vi "_Validate Active Channels.vi"(4 "Negative (F)":bool, 5 "Resolution Type":T1 items=["High/High", "Medium/Medium", "Low/Low", "High/Medium", "High/Low", "Medium/High", "Medium/Low", "Low/High", "Low/Medium"], 6 "error in":errorcluster, 7 "Expt#":i32, 8 "User Res Table (T)":bool=TRUE, 9 "Active Ch":T2[](array[typedef])) -> (0 "error out":errorcluster, 2 "DAC Values":i32[](array[numeric]), 3 "Ch ID":i32[](array[numeric]))   [LabVIEW 2012]
uses:
  Type/_RT Active Ch.ctl
  Type/_RT Res Type.ctl
  _RT Global.vi
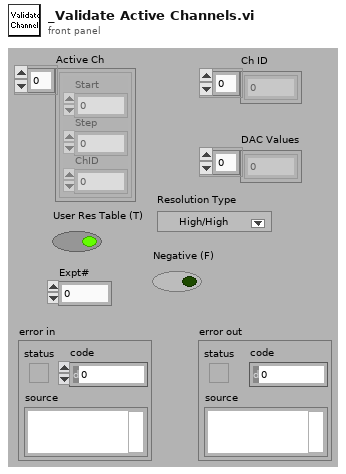
[diagram p1: front panel]
types:
  T1 = typedef "_RT Res Type.ctl" = u16
  T2 = typedef "_RT Active Ch.ctl" = cluster{"Start":i32, "Step":i32, "ChID":i32}
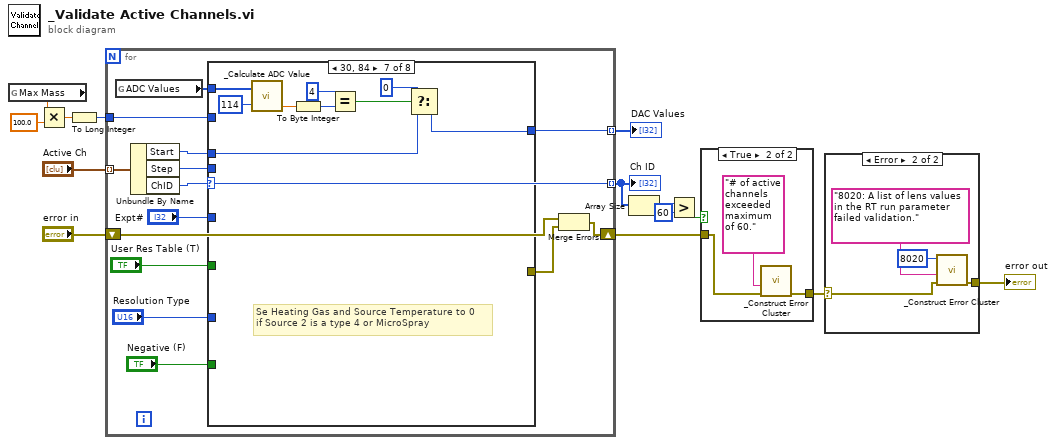
[diagram p0: block diagram]
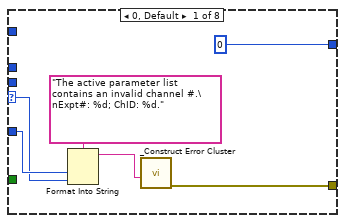
[diagram p4: hidden frame]
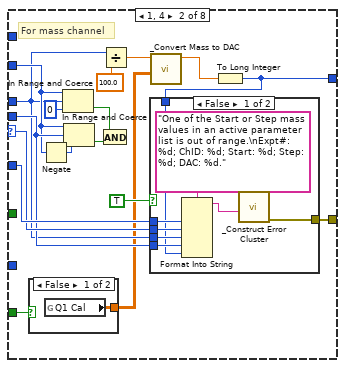
[diagram p5: hidden frame]
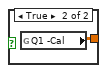
[diagram p6: hidden frame]
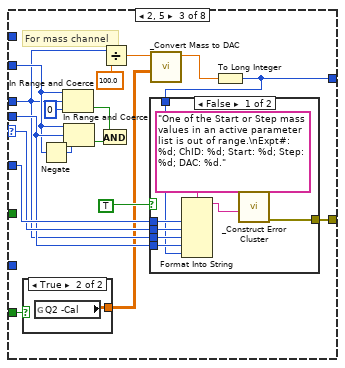
[diagram p8: hidden frame]
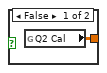
[diagram p9: hidden frame]
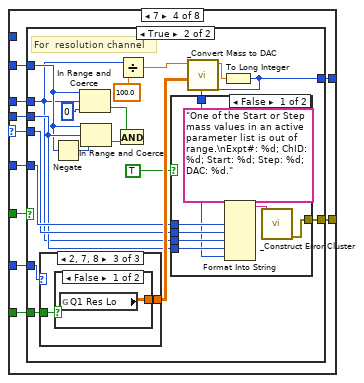
[diagram p11: hidden frame]
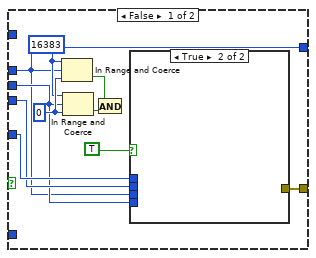
[diagram p12: hidden frame]
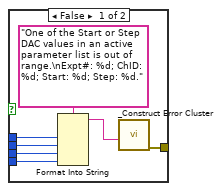
[diagram p13: hidden frame]
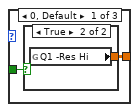
[diagram p14: hidden frame]
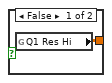
[diagram p15: hidden frame]
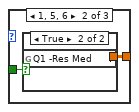
[diagram p16: hidden frame]
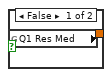
[diagram p17: hidden frame]
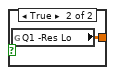
[diagram p18: hidden frame]
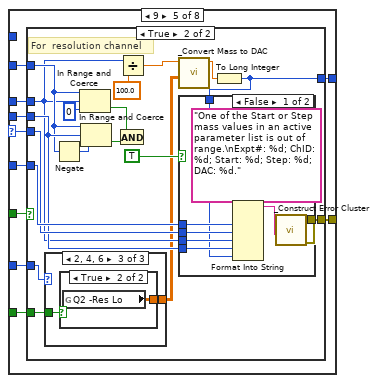
[diagram p20: hidden frame]
diagram:
  n1 = global read "_RT Global.vi" "Max Mass"() -> (w12:dbl)
  n2 = Multiply(x=w12, y=100.0) -> (x*y=w10:dbl)
  n3 = To Long Integer(number=w10) -> (32bit integer=w9:i32)
  n4 = for {
    tunnel: "Active Ch" -> [w28] mode=indexing
    shift-right: [w24] -> w3
    shift-left: "error in" -> [w23]
    tunnel: w9 -> [w25]
    tunnel: [w21] -> w7 mode=indexing
    tunnel: [w20] -> w8 mode=indexing
    n5 = global read "_RT Global.vi" "ADC Values"() -> (w15:i32[])
    n6 = Unbundle By Name(w28) -> ("Start"=w27:i32, "Step"=w26:i32, "ChID"=w21:i32)
    n7 = case shown="30, 84" w21 {
      selector: w21 -> [w31 w43 w70 w91 w156 _ _ w242]
      tunnel: [w34 w48 w75 w93 w158 _ _ w245] -> w22
      tunnel: w27 -> [_ w37 w65 w98 w163 w220 w229 w237]
      tunnel: w26 -> [_ w42 w69 w96 w161 _ _ w241]
      tunnel: w25 -> [_ w38 w67 w97 w162 _ _ _]
      tunnel: [0 ("lower limit") w41 w68 w95 w160 w219 w228 w237] -> w20
      tunnel: "User Res Table (T)" -> [_ _ _ w94 w159 _ _ _]
      tunnel: "Expt#" -> [w32 w44 w71 w92 w157 _ _ w243]
      tunnel: "Resolution Type" -> [_ _ _ w90 w155 _ _ _]
      tunnel: "Negative (F)" -> [_ w36 w63 w89 w154 _ _ _]
      tunnel: w15 -> [_ _ _ _ _ w227 w236 _]
      frame 0, Default {
        n8 = Format Into String(format string="The active parameter list contains an invalid channel #.\nExpt#: %d; ChID: %d.", w32, w31) -> (resulting string=w29:string)  [unwired: 2 in, 1 out]
        n9 = call "_Construct Error Cluster.vi"("reason"=w29) -> ("error out"=w34:errorcluster)  [unwired: 3 in, 3 out]
      }
      frame 1, 4 {
        # "For mass channel"
        n10 = case shown="False" w36 {
          tunnel: [w52 w53] -> w35
          frame False {
            n11 = global read "_RT Global.vi" "Q1 Cal"() -> (w52:dbl[][])
          }
          frame True {
            n12 = global read "_RT Global.vi" "Q1 -Cal"() -> (w53:dbl[][])
          }
        }
        n13 = Negate(x=w38) -> (-x=w40:i32)
        n14 = In Range and Coerce(upper limit=w38, x=w37, lower limit=0) -> (In Range?=w50:bool)  [unwired: 1 out]
        n15 = In Range and Coerce(upper limit=w38, x=w42, lower limit=w40) -> (In Range?=w49:bool)  [unwired: 1 out]
        n16 = And(x=w50, y=w49) -> ()  [unwired: 1 out]
        n17 = Divide(x=w37, y=100.0) -> (x/y=w46:dbl)
        n18 = call "_Convert Mass to DAC.vi"("Calibration Table"=w35, "Mass"=w46) -> ("DAC Value"=w45:dbl)  [unwired: 2 in, 3 out]
        n19 = To Long Integer(number=w45) -> (32bit integer=w41:i32)
        n20 = case shown="False" TRUE {
          tunnel: [w61 _] -> w48
          tunnel: w44 -> [w59 _]
          tunnel: w43 -> [w58 _]
          tunnel: w37 -> [w57 _]
          tunnel: w42 -> [w56 _]
          tunnel: w41 -> [w54 _]
          frame False {
            n21 = Format Into String(format string="One of the Start or Step mass values in an active parameter list is out of range.\nExpt#: %d; ChID: %d; Start: %d; Step: %d; DAC: %d.", w59, w58, w57, w56, w54) -> (resulting string=w55:string)  [unwired: 2 in, 1 out]
            n22 = call "_Construct Error Cluster.vi"("reason"=w55) -> ("error out"=w61:errorcluster)  [unwired: 3 in, 3 out]
          }
          frame True {
          }
        }
      }
      frame 2, 5 {
        # "For mass channel"
        n23 = case shown="True" w63 {
          tunnel: [w79 w80] -> w62
          frame False {
            n24 = global read "_RT Global.vi" "Q2 Cal"() -> (w79:dbl[][])
          }
          frame True {
            n25 = global read "_RT Global.vi" "Q2 -Cal"() -> (w80:dbl[][])
          }
        }
        n26 = Negate(x=w67) -> (-x=w66:i32)
        n27 = In Range and Coerce(upper limit=w67, x=w65, lower limit=0) -> (In Range?=w77:bool)  [unwired: 1 out]
        n28 = In Range and Coerce(upper limit=w67, x=w69, lower limit=w66) -> (In Range?=w76:bool)  [unwired: 1 out]
        n29 = And(x=w77, y=w76) -> ()  [unwired: 1 out]
        n30 = Divide(x=w65, y=100.0) -> (x/y=w73:dbl)
        n31 = call "_Convert Mass to DAC.vi"("Calibration Table"=w62, "Mass"=w73) -> ("DAC Value"=w72:dbl)  [unwired: 2 in, 3 out]
        n32 = To Long Integer(number=w72) -> (32bit integer=w68:i32)
        n33 = case shown="False" TRUE {
          tunnel: [w88 _] -> w75
          tunnel: w71 -> [w86 _]
          tunnel: w70 -> [w85 _]
          tunnel: w65 -> [w84 _]
          tunnel: w69 -> [w83 _]
          tunnel: w68 -> [w81 _]
          frame False {
            n34 = Format Into String(format string="One of the Start or Step mass values in an active parameter list is out of range.\nExpt#: %d; ChID: %d; Start: %d; Step: %d; DAC: %d.", w86, w85, w84, w83, w81) -> (resulting string=w82:string)  [unwired: 2 in, 1 out]
            n35 = call "_Construct Error Cluster.vi"("reason"=w82) -> ("error out"=w88:errorcluster)  [unwired: 3 in, 3 out]
          }
          frame True {
          }
        }
      }
      frame 7 {
        n36 = case shown="True" w94 {
          tunnel: w98 -> [w99 w119]
          tunnel: w97 -> [_ w120]
          tunnel: w96 -> [w101 w123]
          tunnel: [w99 w122] -> w95
          tunnel: [w104 w126] -> w93
          tunnel: w92 -> [w103 w125]
          tunnel: w91 -> [w102 w124]
          tunnel: w90 -> [_ w117]
          tunnel: w89 -> [_ w116]
          frame False {
            w105 = 16383 ("lower limit")
            w108 = 0 ("lower limit")
            n37 = In Range and Coerce(upper limit=w105, x=w99, lower limit=w108) -> (In Range?=w107:bool)  [unwired: 1 out]
            n38 = In Range and Coerce(upper limit=w105, x=w101, lower limit=w108) -> (In Range?=w106:bool)  [unwired: 1 out]
            n39 = And(x=w107, y=w106) -> ()  [unwired: 1 out]
            n40 = case shown="True" TRUE {
              tunnel: [w115 _] -> w104
              tunnel: w103 -> [w114 _]
              tunnel: w102 -> [w113 _]
              tunnel: w99 -> [w112 _]
              tunnel: w101 -> [w111 _]
              frame False {
                n41 = Format Into String(format string="One of the Start or Step  DAC values in an active parameter list is out of range.\nExpt#: %d; ChID: %d; Start: %d; Step: %d.", w114, w113, w112, w111) -> (resulting string=w109:string)  [unwired: 2 in, 1 out]
                n42 = call "_Construct Error Cluster.vi"("reason"=w109) -> ("error out"=w115:errorcluster)  [unwired: 3 in, 3 out]
              }
              frame True {
              }
            }
          }
          frame True {
            # "For  resolution channel"
            n43 = case shown="2, 7, 8" w117 {
              tunnel: [w135 w139 w143] -> w130
              tunnel: w116 -> [w134 w138 w142]
              frame 0, Default {
                n44 = case shown="True" w134 {
                  tunnel: [w136 w137] -> w135
                  frame False {
                    n45 = global read "_RT Global.vi" "Q1 Res Hi"() -> (w136:dbl[][])
                  }
                  frame True {
                    n46 = global read "_RT Global.vi" "Q1 -Res Hi"() -> (w137:dbl[][])
                  }
                }
              }
              frame 1, 5, 6 {
                n47 = case shown="True" w138 {
                  tunnel: [w140 w141] -> w139
                  frame False {
                    n48 = global read "_RT Global.vi" "Q1 Res Med"() -> (w140:dbl[][])
                  }
                  frame True {
                    n49 = global read "_RT Global.vi" "Q1 -Res Med"() -> (w141:dbl[][])
                  }
                }
              }
              frame 2, 7, 8 {
                n50 = case shown="False" w142 {
                  tunnel: [w144 w145] -> w143
                  frame False {
                    n51 = global read "_RT Global.vi" "Q1 Res Lo"() -> (w144:dbl[][])
                  }
                  frame True {
                    n52 = global read "_RT Global.vi" "Q1 -Res Lo"() -> (w145:dbl[][])
                  }
                }
              }
            }
            n53 = Negate(x=w120) -> (-x=w121:i32)
            n54 = In Range and Coerce(upper limit=w120, x=w119, lower limit=0) -> (In Range?=w132:bool)  [unwired: 1 out]
            n55 = In Range and Coerce(upper limit=w120, x=w123, lower limit=w121) -> (In Range?=w131:bool)  [unwired: 1 out]
            n56 = And(x=w132, y=w131) -> ()  [unwired: 1 out]
            n57 = Divide(x=w119, y=100.0) -> (x/y=w128:dbl)
            n58 = call "_Convert Mass to DAC.vi"("Calibration Table"=w130, "Mass"=w128) -> ("DAC Value"=w127:dbl)  [unwired: 2 in, 3 out]
            n59 = To Long Integer(number=w127) -> (32bit integer=w122:i32)
            n60 = case shown="False" TRUE {
              tunnel: [w153 _] -> w126
              tunnel: w125 -> [w151 _]
              tunnel: w124 -> [w150 _]
              tunnel: w119 -> [w149 _]
              tunnel: w123 -> [w148 _]
              tunnel: w122 -> [w146 _]
              frame False {
                n61 = Format Into String(format string="One of the Start or Step mass values in an active parameter list is out of range.\nExpt#: %d; ChID: %d; Start: %d; Step: %d; DAC: %d.", w151, w150, w149, w148, w146) -> (resulting string=w147:string)  [unwired: 2 in, 1 out]
                n62 = call "_Construct Error Cluster.vi"("reason"=w147) -> ("error out"=w153:errorcluster)  [unwired: 3 in, 3 out]
              }
              frame True {
              }
            }
          }
        }
      }
      frame 9 {
        n63 = case shown="True" w159 {
          tunnel: w163 -> [w164 w185]
          tunnel: w162 -> [_ w186]
          tunnel: w161 -> [w166 w189]
          tunnel: [w164 w188] -> w160
          tunnel: [w169 w192] -> w158
          tunnel: w157 -> [w168 w191]
          tunnel: w156 -> [w167 w190]
          tunnel: w155 -> [_ w183]
          tunnel: w154 -> [_ w182]
          frame False {
            w170 = 16383 ("lower limit")
            w173 = 0 ("lower limit")
            n64 = In Range and Coerce(upper limit=w170, x=w164, lower limit=w173) -> (In Range?=w172:bool)  [unwired: 1 out]
            n65 = In Range and Coerce(upper limit=w170, x=w166, lower limit=w173) -> (In Range?=w171:bool)  [unwired: 1 out]
            n66 = And(x=w172, y=w171) -> ()  [unwired: 1 out]
            n67 = case shown="True" TRUE {
              tunnel: [w180 _] -> w169
              tunnel: w168 -> [w179 _]
              tunnel: w167 -> [w178 _]
              tunnel: w164 -> [w177 _]
              tunnel: w166 -> [w176 _]
              frame False {
                n68 = Format Into String(format string="One of the Start or Step  DAC values in an active parameter list is out of range.\nExpt#: %d; ChID: %d; Start: %d; Step: %d.", w179, w178, w177, w176) -> (resulting string=w174:string)  [unwired: 2 in, 1 out]
                n69 = call "_Construct Error Cluster.vi"("reason"=w174) -> ("error out"=w180:errorcluster)  [unwired: 3 in, 3 out]
              }
              frame True {
              }
            }
          }
          frame True {
            # "For  resolution channel"
            n70 = case shown="2, 4, 6" w183 {
              tunnel: [w200 w204 w208] -> w181
              tunnel: w182 -> [w199 w203 w207]
              frame 0, Default {
                n71 = case shown="False" w199 {
                  tunnel: [w201 w202] -> w200
                  frame False {
                    n72 = global read "_RT Global.vi" "Q2 Res Hi"() -> (w201:dbl[][])
                  }
                  frame True {
                    n73 = global read "_RT Global.vi" "Q2 -Res Hi"() -> (w202:dbl[][])
                  }
                }
              }
              frame 1, 3, 8 {
                n74 = case shown="False" w203 {
                  tunnel: [w205 w206] -> w204
                  frame False {
                    n75 = global read "_RT Global.vi" "Q2 Res Med"() -> (w205:dbl[][])
                  }
                  frame True {
                    n76 = global read "_RT Global.vi" "Q2 -Res Med"() -> (w206:dbl[][])
                  }
                }
              }
              frame 2, 4, 6 {
                n77 = case shown="True" w207 {
                  tunnel: [w209 w210] -> w208
                  frame False {
                    n78 = global read "_RT Global.vi" "Q2 Res Lo"() -> (w209:dbl[][])
                  }
                  frame True {
                    n79 = global read "_RT Global.vi" "Q2 -Res Lo"() -> (w210:dbl[][])
                  }
                }
              }
            }
            n80 = Negate(x=w186) -> (-x=w187:i32)
            n81 = In Range and Coerce(upper limit=w186, x=w185, lower limit=0) -> (In Range?=w197:bool)  [unwired: 1 out]
            n82 = In Range and Coerce(upper limit=w186, x=w189, lower limit=w187) -> (In Range?=w196:bool)  [unwired: 1 out]
            n83 = And(x=w197, y=w196) -> ()  [unwired: 1 out]
            n84 = Divide(x=w185, y=100.0) -> (x/y=w194:dbl)
            n85 = call "_Convert Mass to DAC.vi"("Calibration Table"=w181, "Mass"=w194) -> ("DAC Value"=w193:dbl)  [unwired: 2 in, 3 out]
            n86 = To Long Integer(number=w193) -> (32bit integer=w188:i32)
            n87 = case shown="False" TRUE {
              tunnel: [w218 _] -> w192
              tunnel: w191 -> [w216 _]
              tunnel: w190 -> [w215 _]
              tunnel: w185 -> [w214 _]
              tunnel: w189 -> [w213 _]
              tunnel: w188 -> [w211 _]
              frame False {
                n88 = Format Into String(format string="One of the Start or Step mass values in an active parameter list is out of range.\nExpt#: %d; ChID: %d; Start: %d; Step: %d; DAC: %d.", w216, w215, w214, w213, w211) -> (resulting string=w212:string)  [unwired: 2 in, 1 out]
                n89 = call "_Construct Error Cluster.vi"("reason"=w212) -> ("error out"=w218:errorcluster)  [unwired: 3 in, 3 out]
              }
              frame True {
              }
            }
          }
        }
      }
      frame 29, 86 {
        # "Se Heating Gas and Source Temperature to 0\nif Source 1 is a type 4 or MicroSpray"
        n90 = call "_Calculate ADC Value.vi"("ADC Values"=w227, "ADC Channel (64)"=u8 113) -> ("Raw Reading"=w221:sgl)  [unwired: 2 out]
        n91 = To Byte Integer(number=w221) -> (8bit integer=w225:i8)
        n92 = Equal?(x=i8 4, y=w225) -> (x = y?=w223:bool)
        n93 = Select(t=0, s=w223, f=w220) -> (s? t:f=w219:i32)
      }
      frame 30, 84 {
        # "Se Heating Gas and Source Temperature to 0\nif Source 2 is a type 4 or MicroSpray"
        n94 = call "_Calculate ADC Value.vi"("ADC Values"=w236, "ADC Channel (64)"=u8 114) -> ("Raw Reading"=w230:sgl)  [unwired: 2 out]
        n95 = To Byte Integer(number=w230) -> (8bit integer=w234:i8)
        n96 = Equal?(x=i8 4, y=w234) -> (x = y?=w232:bool)
        n97 = Select(t=0, s=w232, f=w229) -> (s? t:f=w228:i32)
      }
      frame 3, 6, 8, 10..28, 31..43, 80..83, 85, 87..94, 200..204 {
        # "For other DAC channels\nand virtual channels (>=200)"
        n98 = In Range and Coerce(upper limit=262143 ("lower limit"), x=w237, lower limit=-262143) -> (In Range?=w247:bool)  [unwired: 1 out]
        n99 = In Range and Coerce(upper limit=2097024 ("lower limit"), x=w241, lower limit=-2097152) -> (In Range?=w246:bool)  [unwired: 1 out]
        n100 = And(x=w247, y=w246) -> ()  [unwired: 1 out]
        n101 = case shown="False" TRUE {
          tunnel: [w255 _] -> w245
          tunnel: w243 -> [w253 _]
          tunnel: w242 -> [w252 _]
          tunnel: w237 -> [w251 _]
          tunnel: w241 -> [w250 _]
          frame False {
            n102 = Format Into String(format string="One of the Start or Step 14-bit DAC values in an active parameter list is out of range.\nExpt#: %d; ChID: %d; Start: %d; Step: %d.", w253, w252, w251, w250) -> (resulting string=w249:string)  [unwired: 2 in, 1 out]
            n103 = call "_Construct Error Cluster.vi"("reason"=w249) -> ("error out"=w255:errorcluster)  [unwired: 3 in, 3 out]
          }
          frame True {
          }
        }
      }
    }
    n104 = Merge Errors(w23, w22) -> (w24:errorcluster)
  }
  "Ch ID" <- w7
  "DAC Values" <- w8
  n105 = Array Size(array=w7) -> (size(s)=w6:i32)
  n106 = Greater?(x=w6, y=60) -> (0:w4:bool)
  n107 = case shown="True" w4 {
    tunnel: w3 -> [w256 w258]
    tunnel: [w256 w257] -> w2
    frame False {
    }
    frame True {
      n108 = call "_Construct Error Cluster.vi"("error in"=w258, "reason"="# of active channels exceeded maximum of 60.") -> ("error out"=w257:errorcluster)  [unwired: 2 in, 3 out]
    }
  }
  n109 = case shown="Error" w2 {
    selector: w2 -> [_ w261]
    tunnel: [_ w260] -> w1
    frame No Error {
    }
    frame Error {
      n110 = call "_Construct Error Cluster.vi"("error in"=w261, "reason"="8020: A list of lens values in the RT run parameter failed validation.", "errorCode"=8020) -> ("error out"=w260:errorcluster)  [unwired: 1 in, 3 out]
    }
  }
  "error out" <- w1
